vi "AI scale.vi"(8 "error in":errorcluster, 11 "Data in":dbl) -> (0 "error out":errorcluster, 3 "Data out":dbl)   [LabVIEW 2015, in "DAQ.lvlib"]
uses:
  DAQ.lvlib
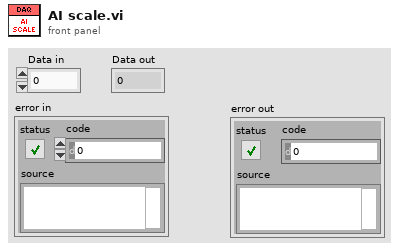
[diagram p1: front panel]
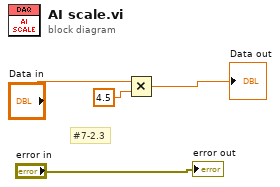
[diagram p0: block diagram]
diagram:
  # "#7-2.3"
  n1 = Multiply(x="Data in", y=4.5) -> (x*y=→"Data out":dbl)
  "error out" <- "error in"
